vi "Encoders(subvi).vi"(0 "Reset Encoders":bool, 5 "Cluster in":T1={FALSE, "Tick Count(uSec)"=0, "Counter Value"=[0, 0, 0, 0], "x-y"=[0, 0, 0, 0]}, 11 "error in (no error)":errorcluster) -> (2 "CM Oikea":dbl, 3 "CM Vasen":dbl, 4 "Tick Count(uSec)":u32 caption="Tick Count(Ticks)", 6 "CM Taka":dbl, 8 "output cluster":T2, 10 "CM Etu":dbl, 13 "Cluster Out":T1, 14 "Updated":bool, 15 "error out":errorcluster)   [LabVIEW 2018]
uses:
  <vilib>/myRIO/Common/Instrument Driver Framework/myRIO v1.0/Encoder/typedefs/Encoder Signal Mode.ctl
  <vilib>/myRIO/Instrument Drivers/Onboard IO/Encoder/typedefs/Encoder Reference.ctl
  <vilib>/myRIO/Common/Instrument Driver Framework/Utilities/typedefs/myRIO Generic Hardware Reference.ctl
  <vilib>/myRIO/Common/Instrument Driver Framework/Utilities/typedefs/Hardware Version Enum.ctl
  <vilib>/myRIO/Common/Instrument Driver Framework/Utilities/typedefs/myRIO v1.0 Reference.ctl
  <vilib>/myRIO/Common/Instrument Driver Framework/Utilities/typedefs/Generic FPGA Reference.ctl
  <vilib>/myRIO/Common/Instrument Driver Framework/myRIO v1.0/Encoder/typedefs/Encoder Channels Enum.ctl
  <vilib>/myRIO/Common/Instrument Driver Framework/myRIO v1.0/Encoder/typedefs/Encoder Configuration v1.0.ctl
  <vilib>/userdefined/High Color/nirio_resource_hc.ctl
  <vilib>/myRIO/Common/Instrument Driver Framework/Utilities/vis/Is FPGA Ref Available.vi
  <vilib>/myRIO/Common/Instrument Driver Framework/myRIO v1.0/Encoder/vis/myRIO v1.1 Open Encoder.vi
  <vilib>/myRIO/Instrument Drivers/Onboard IO/Encoder/vis/Read.vi
  <vilib>/myRIO/Common/Instrument Driver Framework/Utilities/vis/Validate Channels.vi
  <vilib>/myRIO/Common/Instrument Driver Framework/myRIO v1.0/Encoder/vis/myRIO v1.0 Reserve Encoder.vi
  <vilib>/myRIO/Common/Instrument Driver Framework/myRIO v1.0/Encoder/vis/myRIO v1.0 Build MUX Configuration Encoder.vi
  <vilib>/myRIO/Common/Instrument Driver Framework/myRIO v1.0/Resource Manager/vis/myRIO v1.0 Reserve Channel List.vi
  <vilib>/myRIO/Common/Instrument Driver Framework/myRIO v1.0/Resource Manager/vis/myRIO v1.0 Create Configuration List.vi
  <vilib>/myRIO/Common/Instrument Driver Framework/myRIO v1.0/Resource Manager/vis/myRIO v1.0 Reserve Channel.vi
  <vilib>/myRIO/Common/Instrument Driver Framework/myRIO v1.0/Resource Manager/vis/myRIO v1.0 Unreserve Channel.vi
  <vilib>/myRIO/Common/Instrument Driver Framework/myRIO v1.0/Resource Manager/vis/myRIO v1.0 Build Mutex Name.vi
  <vilib>/Utility/VariantDataType/GetNumericInfo.vi
  <vilib>/Utility/error.llb/Error Cluster From Error Code.vi
  <vilib>/myRIO/Common/Instrument Driver Framework/myRIO v1.0/myRIO v1.1 Open.vi
  <vilib>/myRIO/Common/Instrument Driver Framework/Utilities/vis/IO Manager.vi
  <vilib>/myRIO/Common/Instrument Driver Framework/Utilities/vis/Configuration Manager.vi
  <vilib>/myRIO/Common/Instrument Driver Framework/myRIO v1.0/Resource Manager/vis/myRIO v1.0 Configure IO.vi
  <vilib>/myRIO/Common/Instrument Driver Framework/myRIO v1.0/myRIO v1.0 Close.vi
  <vilib>/myRIO/Common/Instrument Driver Framework/myRIO v1.0/Encoder/vis/myRIO v1.0 Configure Encoder.vi
  <vilib>/myRIO/Common/Instrument Driver Framework/myRIO v1.0/Encoder/vis/myRIO v1.0 Read Encoder.vi
  <vilib>/myRIO/Express VI/Onboard IO/Encoder/Encoder Express VI.xnode
  <vilib>/myRIO/Instrument Drivers/Onboard IO/Encoder/vis/myRIO Encoder Open.xnode
  <vilib>/myRIO/Common/Instrument Driver Framework/myRIO v1.0/Encoder/typedefs/Encoder Count Direction Enum.ctl
  <vilib>/rvi/Arithmetic/AddSubMult/XNode/nirviSatArithmetic.xnode
  <vilib>/myRIO/Instrument Drivers/Onboard IO/Encoder/Encoder.lvlib
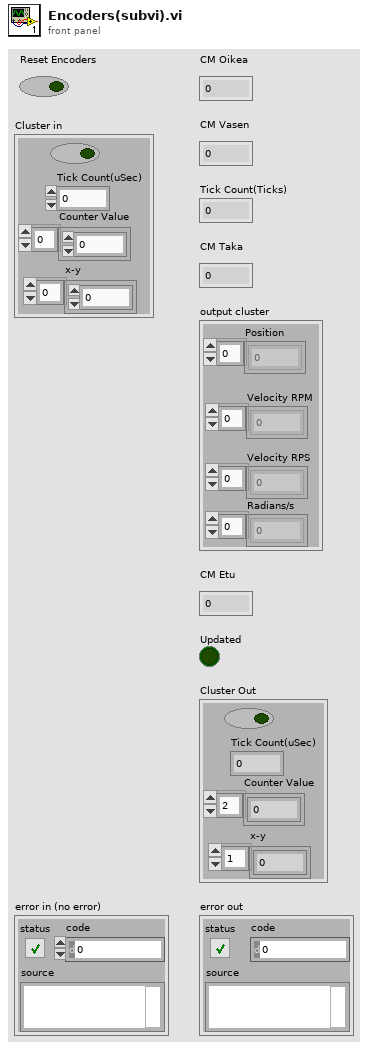
[diagram p1: front panel]
types:
  T1 = cluster{bool, "Tick Count(uSec)":u32, "Counter Value":i32[], "x-y":i32[]}
  T2 = cluster{"Position":i32[], "Velocity RPM":dbl[], "Velocity RPS":dbl[], "Radians/s":dbl[]}
  T3 = cluster{"Counter Value":i32[], dbl[], dbl[], dbl[]}
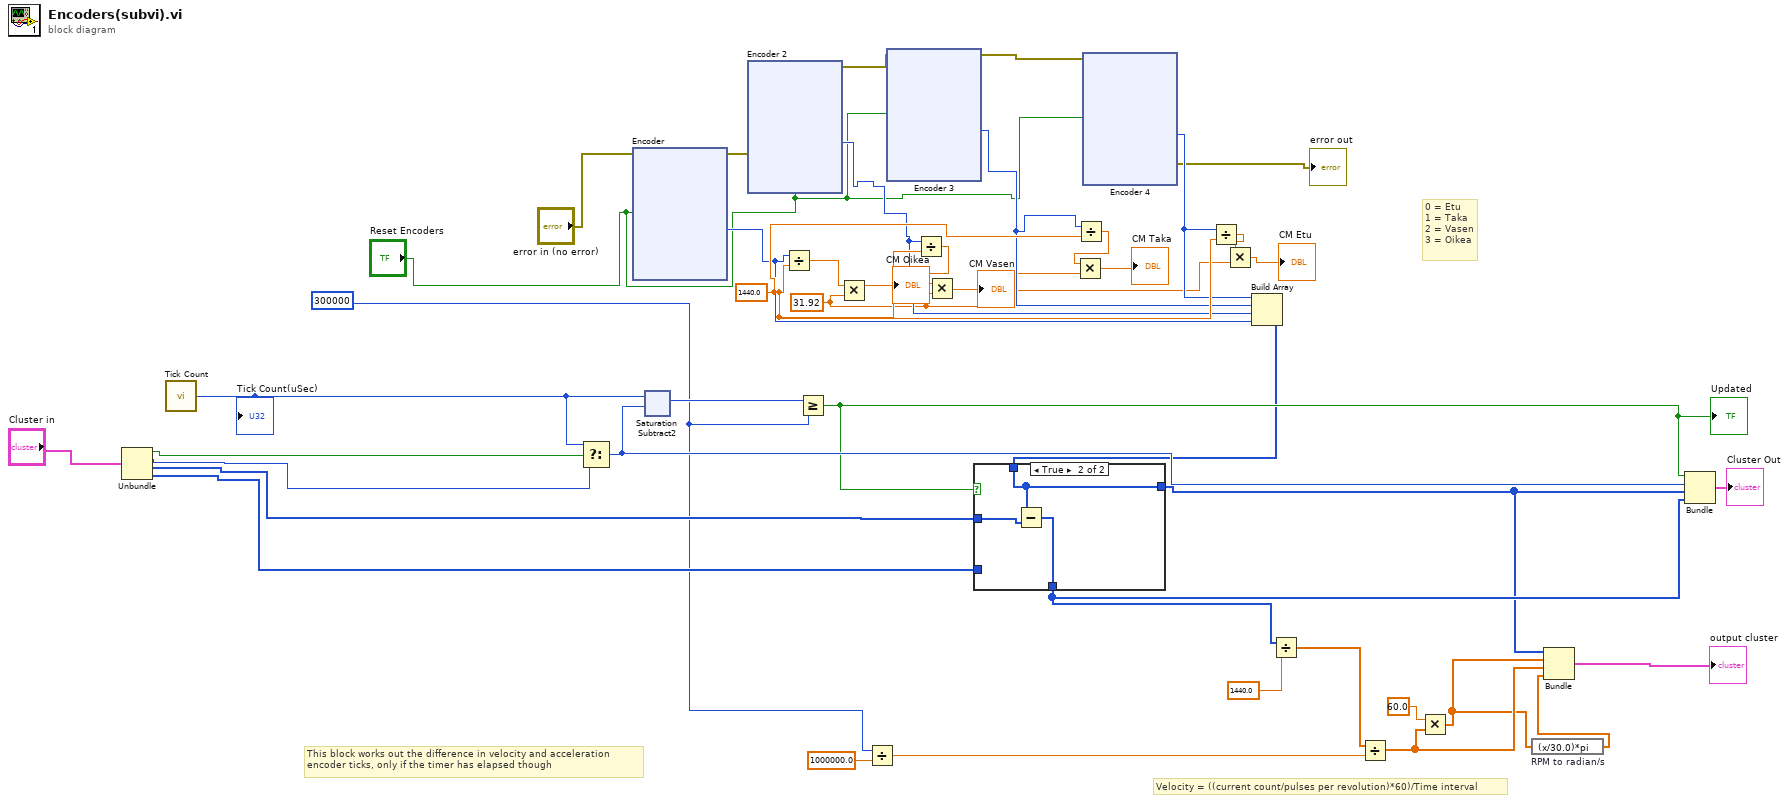
[diagram p0: block diagram]
diagram:
  w43 = 1440.0
  w34 = 31.92
  w3 = 300000
  # "0 = Etu\n1 = Taka\n2 = Vasen\n3 = Oikea"
  # "Velocity = ((current count/pulses per revolution)*60)/Time interval"
  # "This block works out the difference in velocity and acceleration \nencoder ticks, only if the timer has elapsed though"
  n1 = Unbundle("Cluster in") -> (w13:bool, "Tick Count(uSec)"=w12:u32, "Counter Value"=w11:i32[], "x-y"=w10:i32[])
  n2 = call "Tick Count"() -> ("Tick Count(uSec)"=w23:u32)
  "Tick Count(uSec)" <- w23
  n3 = Select(t=w23, s=w13, f=w12) -> (s? t:f=w22:u32)
  n4 = xnode "Encoder"("Reset Counter"="Reset Encoders", "error in (no error)"="error in (no error)") -> ("Counter Value"=w31:i32, "error out"=w17:errorcluster)  [unwired: 2 out]
  n5 = xnode ("Saturation Subtract2")("x"=w23, "y"=w22) -> ("x-y"=w18:u32)
  n6 = xnode "Encoder 2"("Reset Counter"="Reset Encoders", "error in (no error)"=w17) -> ("Counter Value"=w39:i32, "error out"=w6:errorcluster)  [unwired: 2 out]
  n7 = Divide(x=w31, y=w43) -> (x/y=w32:dbl)
  n8 = Greater Or Equal?(x=w18, y=w3) -> (x >= y?=w21:bool)
  "Updated" <- w21
  n9 = Multiply(x=w32, y=w34) -> (x*y=→"CM Oikea":dbl)
  n10 = Divide(x=w3, y=1000000.0) -> (x/y=w25:dbl)
  n11 = xnode "Encoder 3"("Reset Counter"="Reset Encoders", "error in (no error)"=w6) -> ("Counter Value"=w40:i32, "error out"=w5:errorcluster)  [unwired: 2 out]
  n12 = Divide(x=w39, y=w43) -> (x/y=w38:dbl)
  n13 = Multiply(x=w38, y=w34) -> (x*y=→"CM Vasen":dbl)
  n14 = Divide(x=w40, y=w43) -> (x/y=w37:dbl)
  n15 = Multiply(x=w37, y=w34) -> (x*y=→"CM Taka":dbl)
  n16 = xnode "Encoder 4"("Reset Counter"="Reset Encoders", "error in (no error)"=w5) -> ("Counter Value"=w42:i32, "error out"=→"error out":errorcluster)  [unwired: 2 out]
  n17 = Divide(x=w42, y=w43) -> (x/y=w36:dbl)
  n18 = Multiply(x=w36, y=w34) -> (x*y=→"CM Etu":dbl)
  n19 = Build Array(w42, w40, w39, w31) -> (w16:i32[])
  n20 = case shown="True" w21 {
    tunnel: w11 -> [w44 w48]
    tunnel: [w45 w47] -> w26
    tunnel: w10 -> [w45 _]
    tunnel: [w44 w46] -> w24
    tunnel: w16 -> [_ w46]
    frame False {
    }
    frame True {
      n21 = Subtract(x=w46, y=w48) -> (x-y=w47:i32[])
    }
  }
  n22 = Divide(x=w26, y=1440.0) -> (x/y=w27:dbl[])
  n23 = Divide(x=w27, y=w25) -> (x/y=w28:dbl[])
  n24 = Multiply(x=60.0 ("y"), y=w28) -> (x*y=w9:dbl[])
  n25 = expression code="(x/30.0)*pi" "RPM to radian/s"(w9) -> (w8:dbl[])
  n26 = Bundle("Counter Value"=w24, w9, w28, w8) -> (→"output cluster":T3)  [unwired: 1 in]
  n27 = Bundle(w21, "Tick Count(uSec)"=w22, "Counter Value"=w24, "x-y"=w26) -> (→"Cluster Out":T1)  [unwired: 1 in]
